vi "Example_Fitting.vi"() -> ()   [LabVIEW 2012]
panel:
  out "Gaussian":dbl[][](graph)
  out "Lorentzian":dbl[][](graph)
  out "Intensity Graph":dbl[][](graph)
  in  "a":dbl[](array[numeric])
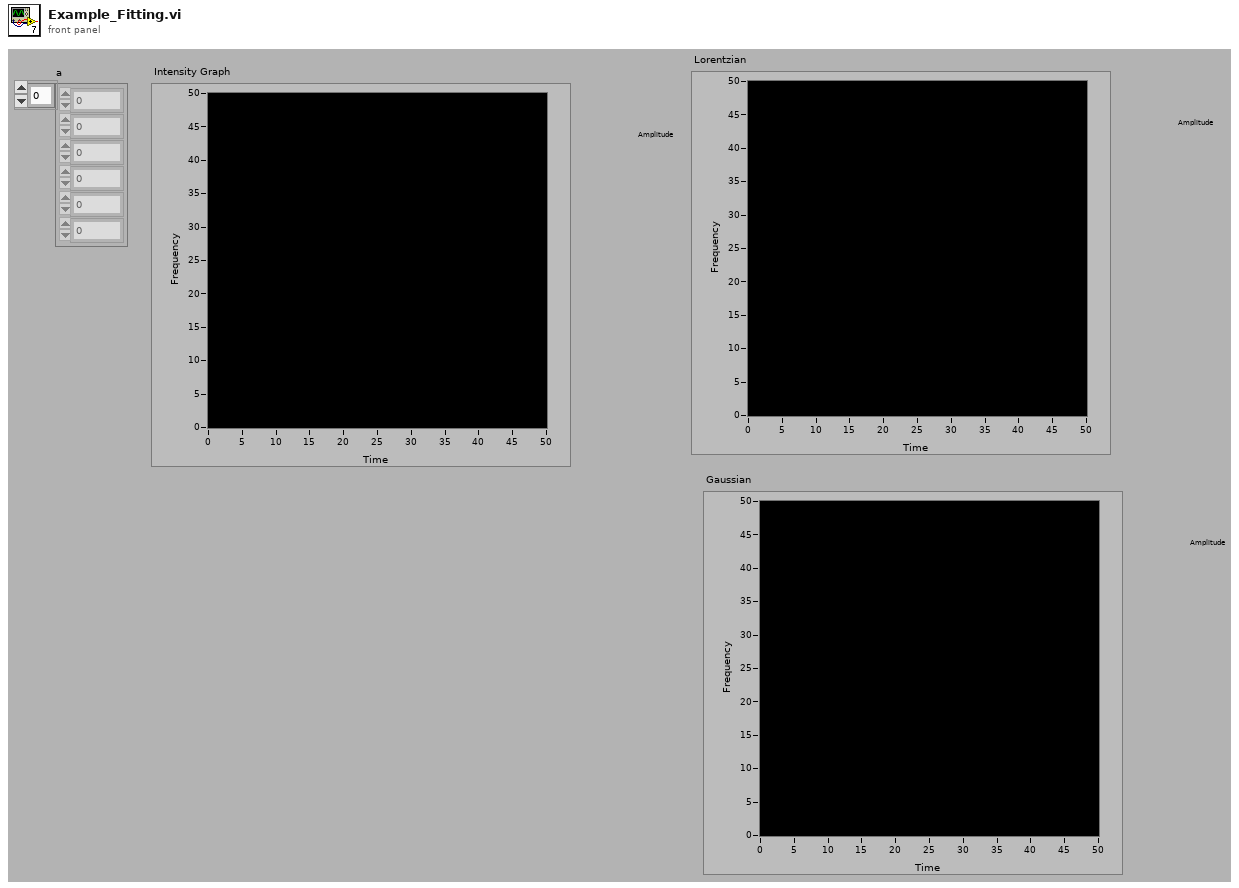
[diagram p1: front panel]
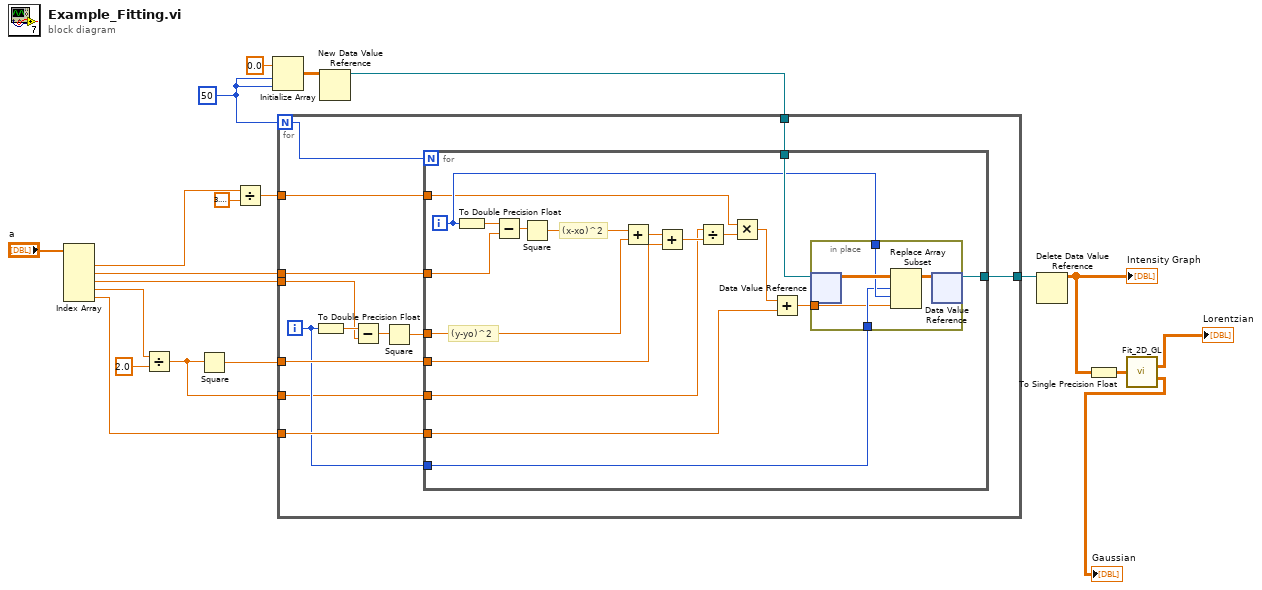
[diagram p0: block diagram]
diagram:
  w5 = 50
  n1 = Index Array(array="a") -> (element #1=w11:dbl, element #2=w19:dbl, element #3=w18:dbl, element #4=w9:dbl, element #5=w13:dbl)  [unwired: 5 in]
  n2 = Divide(x=w9, y=2.0) -> (x/y=w6:dbl)
  n3 = Square(x=w6) -> (x^2=w7:dbl)
  n4 = Divide(x=w11, y=3.141592653589793) -> (x/y=w10:dbl)
  n5 = Initialize Array(0.0 ("element"), w5, w5) -> (w16:dbl[][])
  n6 = New Data Value Reference(data value=w16) -> (data value reference=w15:refnum<data-value>)  [unwired: 1 in, 1 out]
  n7 = for {
    N: w5 -> [w33]
    tunnel: w10 -> [w32]
    tunnel: w19 -> [w31]
    tunnel: w18 -> [w28]
    tunnel: w13 -> [w30]
    tunnel: w7 -> [w25]
    tunnel: w15 -> [w24]
    tunnel: [w22] -> w14
    tunnel: w6 -> [w21]
    i -> [w23]
    n8 = To Double Precision Float(number=w23) -> (double precision float=w29:dbl)
    n9 = Subtract(x=w29, y=w28) -> (x-y=w27:dbl)
    n10 = Square(x=w27) -> (x^2=w26:dbl)
    n11 = for {
      N: w33 -> [_]
      tunnel: w32 -> [w37]
      tunnel: w31 -> [w50]
      tunnel: w30 -> [w35]
      tunnel: w26 -> [w40]
      tunnel: w25 -> [w42]
      tunnel: w24 -> [w48]
      tunnel: w23 -> [w46]
      tunnel: [w45] -> w22
      tunnel: w21 -> [w39]
      i -> [w47]
      # "(y-yo)^2"
      # "(x-xo)^2"
      n12 = To Double Precision Float(number=w47) -> (double precision float=w51:dbl)
      n13 = Subtract(x=w51, y=w50) -> (x-y=w49:dbl)
      n14 = Square(x=w49) -> (x^2=w41:dbl)
      n15 = Add(x=w41, y=w40) -> (x+y=w44:dbl)
      n16 = Add(x=w44, y=w42) -> (x+y=w43:dbl)
      n17 = Divide(x=w39, y=w43) -> (x/y=w38:dbl)
      n18 = Multiply(x=w37, y=w38) -> (x*y=w36:dbl)
      n19 = Add(x=w36, y=w35) -> (x+y=w34:dbl)
      n20 = in-place {
        in-place-border: w47 -> [w54]
        in-place-border: w46 -> [w53]
        in-place-border: w34 -> [w52]
        n21 = in-place-dvr #1(w48) -> (w56:dbl[][])  [unwired: 1 out]
        n22 = Replace Array Subset(array=w56, new element=w52, index (row)=w53, index (col)=w54) -> (w55:dbl[][])
        n23 = in-place-dvr #1(w55) -> (w45:refnum<data-value>)  [unwired: 1 out]
      }
    }
  }
  n24 = Delete Data Value Reference(data value reference=w14) -> (data value=w4:dbl[][])  [unwired: 1 in, 1 out]
  "Intensity Graph" <- w4
  n25 = To Single Precision Float(number=w4) -> (single precision float=w3:sgl[][])
  n26 = call "Fit_2D_GL.vi"("Image IN"=w3) -> ("Lorentzian Image"=→"Lorentzian":dbl[][], "Gaussian Image"=→"Gaussian":dbl[][])  [unwired: 10 in, 3 out]
